vi "Query Actual Temperature 9620.vi"(8 "error in (no error)":errorcluster, 11 "VISA resource name":refnum<visa-resource-name>="COM3") -> (0 "error out":errorcluster, 2 "Current actual temperature":dbl, 3 "VISA resource name out":refnum<visa-resource-name>)   [LabVIEW 2017]
panel:
  out "Command string":string="S"
  out "read buffer":string
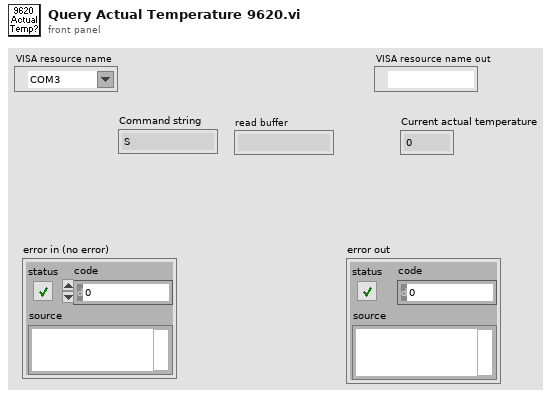
[diagram p1: front panel]
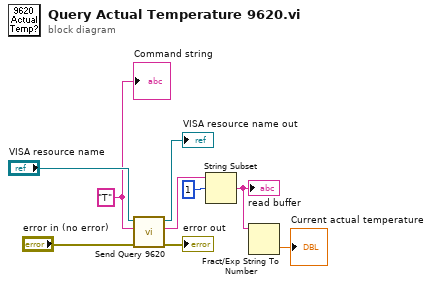
[diagram p0: block diagram]
diagram:
  w4 = "T"
  n1 = call "Send Query 9620.vi"("error in (no error)"="error in (no error)", "Query"=w4, "VISA resource name"="VISA resource name") -> ("error out"=→"error out":errorcluster, "read buffer"=w1:string, "VISA resource name out"=→"VISA resource name out":refnum<visa-resource-name>)  [unwired: 6 in]
  n2 = String Subset(string=w1, offset (0)=1) -> (substring=w3:string)  [unwired: 1 in]
  "read buffer" <- w3
  n3 = Fract/Exp String To Number(string=w3) -> (number=→"Current actual temperature":dbl)  [unwired: 3 in, 1 out]
  "Command string" <- w4
